vi "VCS Find SubDevice Communication Settings.vi"(0 "axis in":cluster{"keyHandle":u32, "nodeId":u16}={"keyHandle"=0, "nodeId"=1}, 1 "pBaudrate":u32, 3 "DialogMode":i32(ring) items=["Progress Dialog", "Progress and Confirmation Dialog", "Confirmation Dialog", "No Dialog"], 5 "pDeviceName":string, 7 "SizeName":u16, 9 "pProtocolStackName":string, 11 "error in (no error)":errorcluster) -> (4 "axis out":cluster{"keyHandle":u32, "nodeId":u16}={"keyHandle"=0, "nodeId"=1}, 6 "pDeviceName out":string, 10 "pProtocolStackName out":string, 12 "pBaudrate out":u32, 15 "error out":errorcluster)   [LabVIEW 2017, in "maxonEPOS.lvlib"]
doc: "<B>VCS_FindSubDeviceCommunicationSettings</B> searches the subdevice communication setting parameters. Parameters can be defined to accelerate the process. The search will be terminated as the first device is found."
uses:
  Examples/maxonEPOS.lvlib
  SSI_Tool/InstrumentsInterfaces/Motordriver/maxon EPOS/Resources/EposCmd64.dll
  SSI_Tool/InstrumentsInterfaces/Motordriver/maxon EPOS/Resources/EposCmd.dll
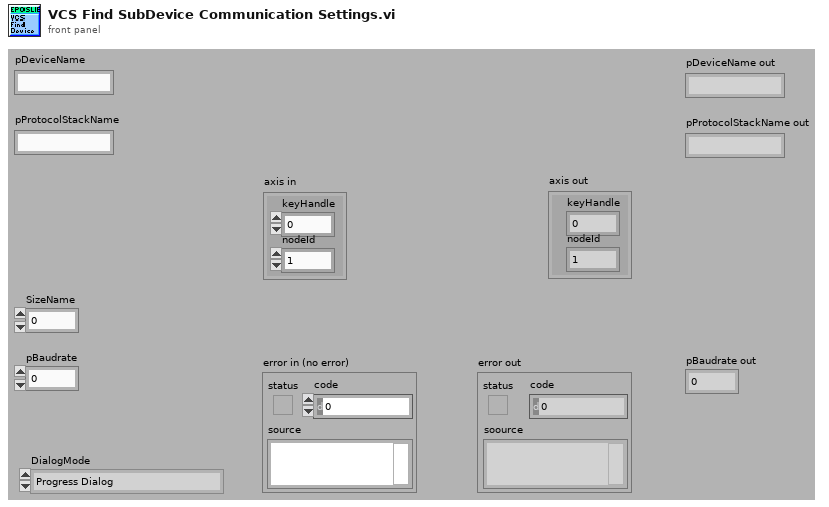
[diagram p1: front panel]
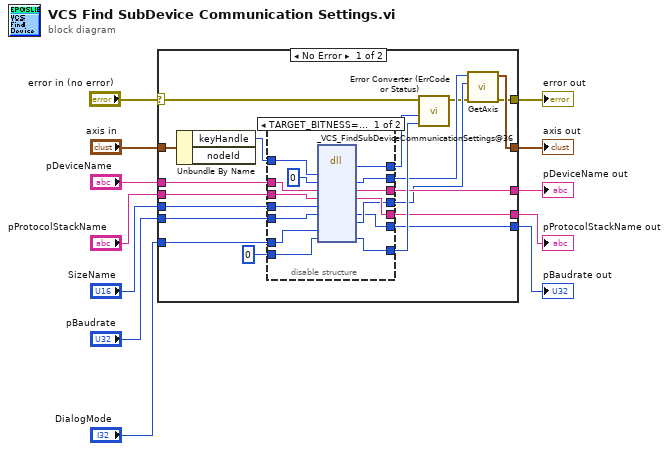
[diagram p0: block diagram]
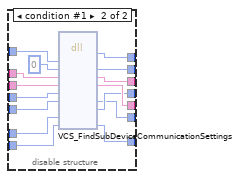
[diagram p2: hidden frame]
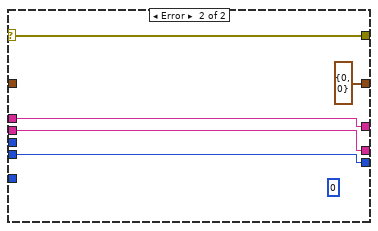
[diagram p3: hidden frame]
diagram:
  n1 = case shown="No Error" "error in (no error)" {
    selector: "error in (no error)" -> [w30 w66]
    tunnel: "axis in" -> [w31 _]
    tunnel: [w13 w66] -> w11
    tunnel: "pDeviceName" -> [w28 w65]
    tunnel: [w24 w65] -> w8
    tunnel: [w23 w64] -> w7
    tunnel: [w22 w63] -> w6
    tunnel: "pProtocolStackName" -> [w21 w64]
    tunnel: "SizeName" -> [w20 _]
    tunnel: "pBaudrate" -> [w19 w63]
    tunnel: "DialogMode" -> [w18 _]
    tunnel: [w15 cluster{"keyHandle":u32, "nodeId":u16} {"keyHandle"=0, "nodeId"=0} ("axis out")] -> w1
    frame No Error {
      n2 = Unbundle By Name(w31) -> ("keyHandle"=w27:u32)  [unwired: 1 out]
      n3 = disable-structure shown="TARGET_BITNESS==32, Standard" {
        disable-tunnel: u32 0 ("pErrorCode") -> [w33 w61]
        disable-tunnel: w28 -> [w46 w60]
        disable-tunnel: w27 -> [w36 w49]
        disable-tunnel: [w45 w59] -> w26
        disable-tunnel: [w44 w58] -> w25
        disable-tunnel: [w43 w57] -> w24
        disable-tunnel: [w42 w56] -> w23
        disable-tunnel: [w41 w55] -> w16
        disable-tunnel: [w40 w54] -> w22
        disable-tunnel: w21 -> [w39 w53]
        disable-tunnel: w20 -> [w38 w52]
        disable-tunnel: w19 -> [w37 w51]
        disable-tunnel: w18 -> [w32 w50]
        disable-tunnel: [w35 w47] -> w17
        frame condition #0 (active) {
          n4 = dll-call lib="C:/workspace/project/scancon/sw/SSI_Tool/InstrumentsInterfaces/Motordriver/maxon EPOS/Resources/EposCmd.dll" fn="_VCS_FindSubDeviceCommunicationSettings@36"("deviceHandle"=w36, "pKeyHandle"=u32 0, "pDeviceName"=w46, "pProtocolStackName"=w39, "SizeName"=w38, "pBaudrate"=w37, "ShowMsg"=w32, "pErrorCode"=w33) -> ("Rückgabetyp"=w44:i32, "pKeyHandle"=w35:u32, "pDeviceName"=w43:string, "pProtocolStackName"=w42:string, "pBaudrate"=w40:u32, "pNodeId"=w41:u16, "pErrorCode"=w45:u32)  [unwired: 7 in, 2 out]
        }
        frame condition #1 {
          n5 = dll-call lib="C:/Sources/LabView/maxon EPOS/Resources/EposCmd64.dll" fn="VCS_FindSubDeviceCommunicationSettings"("deviceHandle"=w49, "pKeyHandle"=u32 0, "pDeviceName"=w60, "pProtocolStackName"=w53, "SizeName"=w52, "pBaudrate"=w51, "ShowMsg"=w50, "pErrorCode"=w61) -> ("return type"=w58:i32, "pKeyHandle"=w47:u32, "pDeviceName"=w57:string, "pProtocolStackName"=w56:string, "pBaudrate"=w54:u32, "pNodeId"=w55:u16, "pErrorCode"=w59:u32)  [unwired: 7 in, 2 out]
        }
      }
      n6 = call "Error Converter (ErrCode or Status).vi"("error code"=w26, "return type"=w25, "error in (no error)"=w30) -> ("error out"=w14:errorcluster)  [unwired: 7 in]
      n7 = call "GetAxis.vi"("error in (no error)"=w14, "nodeId"=w16, "keyHandle in"=w17) -> ("error out"=w13:errorcluster, "axis out"=w15:cluster{"keyHandle":u32, "nodeId":u16})  [unwired: 7 in]
    }
    frame Error {
      (unwired) u16 0 ("pNodeId")
    }
  }
  "pDeviceName out" <- w8
  "pProtocolStackName out" <- w7
  "pBaudrate out" <- w6
  "error out" <- w11
  "axis out" <- w1
